vi "均匀性均值差值.vi"(9 "位置":enum16{"A", "B", "C", "D", "E", "F", "G", "H"}(ring), 11 "均匀性表格":string[][](table)=[["A", "O", "E", "O"], ["", "", "", ""], ["", "", "", ""], ["", "", "", ""], ["", "", "", ""], ["", "", "", ""], ["", "", "", ""], ["B", "O", "F", "O"], ["", "", "", ""], ["", "", "", ""], ["", "", "", ""], ["", "", "", ""], ["", "", "", ""], ["", "", "", ""], ["C", "O", "G", "O"], ["", "", "", ""], ["", "", "", ""], ["", "", "", ""], ["", "", "", ""], ["", "", "", ""], ["", "", "", ""], ["D", "O", "H", "O"], ["", "", "", ""], ["", "", "", ""], ["", "", "", ""], ["", "", "", ""], ["", "", "", ""], ["", "", "", ""], ["", "", "", ""], ["", "", "", ""]]) -> (3 "输出数组":string[][](array[string]))   [LabVIEW 2015]
uses:
  <vilib>/Analysis/baseanly.llb/Mean (DBL).vi
  <vilib>/Analysis/NI_AALBase.lvlib
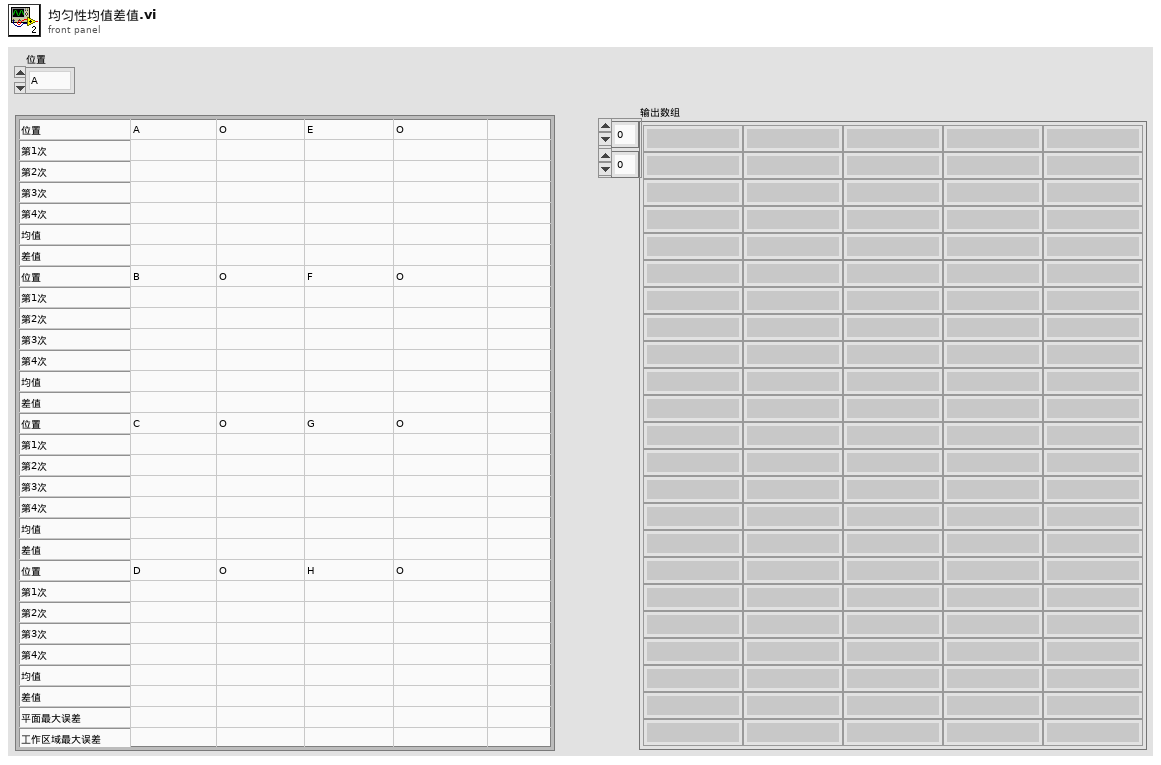
[diagram p1: front panel]
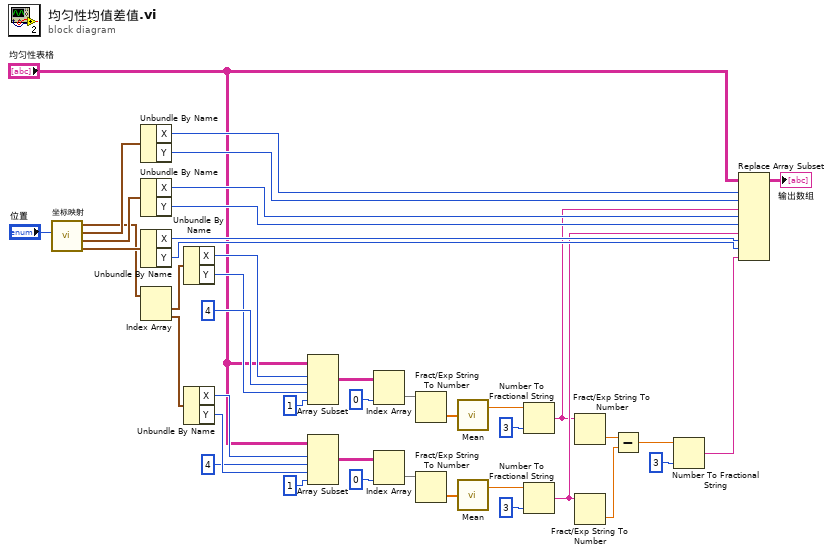
[diagram p0: block diagram]
diagram:
  n1 = call "坐标映射.vi"("位置"="位置") -> ("差值坐标"=w35:cluster{"X":i32, "Y":i32}, "O均值坐标"=w38:cluster{"X":i32, "Y":i32}, "位置均值坐标"=w41:cluster{"X":i32, "Y":i32}, "位置坐标"=w27:cluster{"X":i32, "Y":i32}[])  [unwired: 7 in]
  n2 = Unbundle By Name(w41) -> ("X"=w40:i32, "Y"=w39:i32)
  n3 = Unbundle By Name(w38) -> ("X"=w37:i32, "Y"=w36:i32)
  n4 = Unbundle By Name(w35) -> ("X"=w34:i32, "Y"=w33:i32)
  n5 = Index Array(array=w27) -> (element #1=w26:cluster{"X":i32, "Y":i32}, element #2=w25:cluster{"X":i32, "Y":i32})  [unwired: 2 in]
  n6 = Unbundle By Name(w26) -> ("X"=w24:i32, "Y"=w23:i32)
  n7 = Unbundle By Name(w25) -> ("X"=w22:i32, "Y"=w21:i32)
  n8 = Array Subset(array="均匀性表格", index (row)=w24, length (row)=4 ("长度"), index (col)=w23, length (col)=1 ("长度")) -> (w29:string[][])
  n9 = Array Subset(array="均匀性表格", index (row)=w22, length (row)=4 ("长度"), index (col)=w21, length (col)=1 ("长度")) -> (w8:string[][])
  n10 = Index Array(array=w29, index (col)=0 ("索引 (行)")) -> (element=w17:string[])  [unwired: 1 in]
  n11 = Index Array(array=w8, index (col)=0 ("索引 (行)")) -> (element=w10:string[])  [unwired: 1 in]
  n12 = Fract/Exp String To Number(string=w17) -> (number=w16:dbl[])  [unwired: 3 in, 1 out]
  n13 = Fract/Exp String To Number(string=w10) -> (number=w11:dbl[])  [unwired: 3 in, 1 out]
  n14 = call-poly <vilib>:"Mean.vi"("X"=w16) -> ("mean"=w15:dbl)  [unwired: 1 out]
  n15 = call-poly <vilib>:"Mean.vi"("X"=w11) -> ("mean"=w12:dbl)  [unwired: 1 out]
  n16 = Number To Fractional String(number=w15, precision (6)=i16 3 ("精度(6)")) -> (F-format string=w6:string)  [unwired: 2 in]
  n17 = Number To Fractional String(number=w12, precision (6)=i16 3 ("精度(6)")) -> (F-format string=w7:string)  [unwired: 2 in]
  n18 = Fract/Exp String To Number(string=w6) -> (number=w5:dbl)  [unwired: 3 in, 1 out]
  n19 = Fract/Exp String To Number(string=w7) -> (number=w4:dbl)  [unwired: 3 in, 1 out]
  n20 = Subtract(x=w5, y=w4) -> (x-y=w2:dbl)
  n21 = Number To Fractional String(number=w2, precision (6)=i16 3 ("精度(6)")) -> (F-format string=w1:string)  [unwired: 2 in]
  n22 = Replace Array Subset(array="均匀性表格", new element #1=w6, index (row) #1=w40, index (col) #1=w39, new element #2=w7, index (row) #2=w37, index (col) #2=w36, new element #3=w1, index (row) #3=w34, index (col) #3=w33) -> (→"输出数组":string[][])
